vi "mod_Plot FSK Eye Diagram.vi"(0 "Input Complex Waveform":T1={"t0"=0.0, "dt"=1.0, "Y"=[]} {"Y" format="%.3f"; "dt" format="%^.2e"; "t0" format="%.4f"}, 1 "Rx Eye Diagram":refnum<vi>, 2 "autoscale":bool, 5 "eye length":i32=3, 7 "Symbol Rate, Hz":dbl format="%.2f", 9 "matched filter coefficients":dbl[](array[numeric])=[1.0] format="%^.2g", 11 "error in (no error)":errorcluster, 12 "Reset?":bool) -> (4 "FSK Eye Diagram":cluster{"t0":dbl, "dt":dbl, "Y":dbl[]}[](array[cluster]) {"Y" format="%.2f"; "dt" format="%.2f"; "t0" format="%.2f"}, 6 "output FM demodulated waveform":waveform(dbl), 15 "error out":errorcluster)   [LabVIEW 2020, in "niDMT.lvlib"]
uses:
  <vilib>/addons/Modulation/niDMT.lvlib
  <vilib>/addons/Modulation/Analog/controls/Complex Data Waveform.ctl
  <vilib>/addons/Modulation/Digital/General/MT Apply Matched Filter (Generic).vi
  <vilib>/addons/Modulation/Digital/General/MT Format Eye Diagram (WDT).vi
  <vilib>/addons/Modulation/niAMT.lvlib
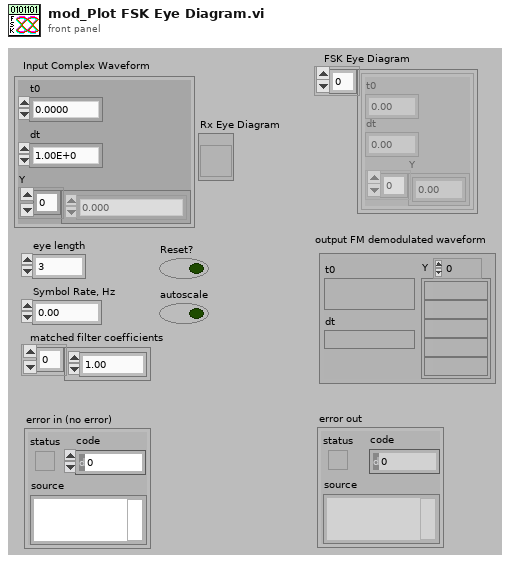
[diagram p1: front panel]
types:
  T1 = typedef "niAMT.lvlib/Complex Data Waveform.ctl" = cluster{"t0":dbl, "dt":dbl, "Y":cdb[]}
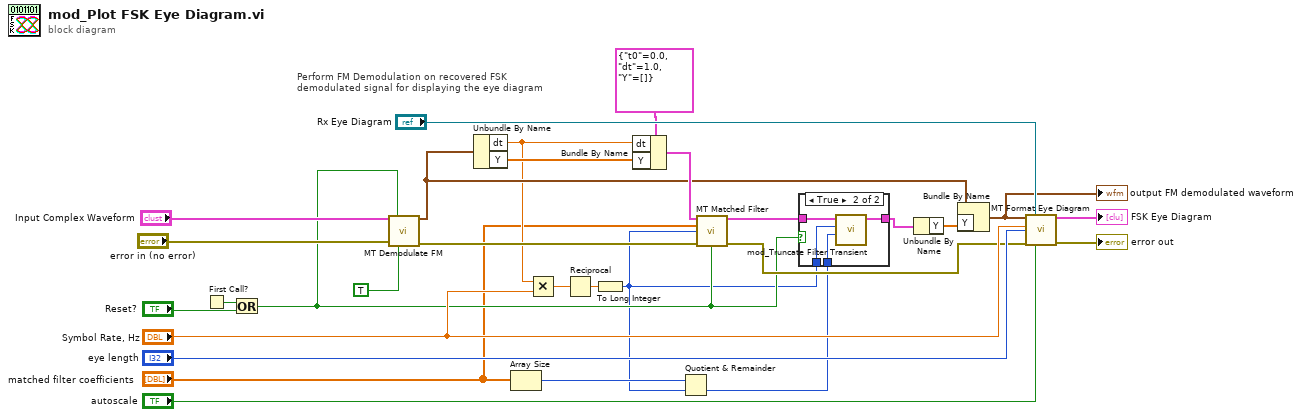
[diagram p0: block diagram]
diagram:
  # "Perform FM Demodulation on recovered FSK\ndemodulated signal for displaying the eye diagram"
  n1 = First Call?() -> (First Call?: T/F=w11:bool)
  n2 = Or(x=w11, y="Reset?") -> (x .or. y?=w6:bool)
  n3 = call <vilib>:"MT Demodulate FM.vi"("FM modulated waveform"="Input Complex Waveform", "reset? (F)"=w6, "error in (no error)"="error in (no error)", "remove transient when reset? (F)"=TRUE ("remove transient\nwhen reset? (F)")) -> ("FM demodulated waveform"=w17:waveform(dbl), "error out"=w15:errorcluster)  [unwired: 2 in, 8 out]
  n4 = Unbundle By Name(w17) -> ("dt"=w13:dbl, "Y"=w20:dbl[])
  n5 = Array Size(array="matched filter coefficients") -> (size(s)=w3:i32)
  n6 = Multiply(x=w13, y="Symbol Rate, Hz") -> (x*y=w12:dbl)
  n7 = Reciprocal(x=w12) -> (1/x=w5:dbl)
  n8 = To Long Integer(number=w5) -> (32bit integer=w2:i32)
  n9 = Bundle By Name(cluster=cluster{"t0":dbl, "dt":dbl, "Y":cdb[]} {"t0"=0.0, "dt"=1.0, "Y"=[]} ("input complex waveform"), "dt"=w13, "Y"=w20) -> (w19:cluster{"t0":dbl, "dt":dbl, "Y":cdb[]})
  n10 = Quotient & Remainder(x=w3, y=w2) -> (floor(x/y)=w1:i32)  [unwired: 1 out]
  n11 = call-poly <vilib>:"MT Matched Filter.vi"("input complex waveform"=w19, "matched filter coefficients"="matched filter coefficients", "samples per symbol (16)"=w2, "error in (no error)"=w15, "reset? (T)"=w6) -> ("output complex waveform"=w9:T1, "error out"=w7:errorcluster)  [unwired: 9 out]
  n12 = case shown="True" w6 {
    tunnel: w9 -> [w30 w34]
    tunnel: [w30 w33] -> w8
    tunnel: w2 -> [_ w32]
    tunnel: w1 -> [_ w31]
    frame False {
    }
    frame True {
      n13 = call <vilib>:"mod_Truncate Filter Transient.vi"("filter length (sym)"=w31, "samples/symbol"=w32, "input complex waveform"=w34) -> ("output complex waveform"=w33:T1)  [unwired: 8 out]
    }
  }
  n14 = Unbundle By Name(w8) -> ("Y"=w18:cdb[])
  n15 = Bundle By Name(cluster=w17, "Y"=w18) -> (w16:waveform(dbl))
  "output FM demodulated waveform" <- w16
  n16 = call-poly <vilib>:"MT Format Eye Diagram.vi"("waveform"=w16, "eye diagram reference"="Rx Eye Diagram", "symbol rate (Hz)"="Symbol Rate, Hz", "eye length"="eye length", "error in (no error)"=w7, "autoscale"="autoscale") -> ("eye diagram"=→"FSK Eye Diagram":cluster{"t0":dbl, "dt":dbl, "Y":dbl[]}[], "error out"=→"error out":errorcluster)  [unwired: 8 out]
